vi "configuration UI.vi"() -> ()   [LabVIEW 2013, in "UI Reference editor node.lvclass"]
uses:
  UI Reference editor node.lvclass
  <vilib>/CEF_TreeControl/Node/NodeRef.ctl
  <vilib>/CEF_TreeControl/Node/NISE_CEF_Node.lvclass
  <vilib>/NI/AMC/Message Queue.ctl
  <vilib>/NI/AMC/Message.ctl
  <vilib>/NI/Tools/Keyed Array/KeyedArray.ctl
  <vilib>/CEF_TreeControl/Node/UserEventRef.ctl
  <vilib>/CEF_TreeControl/Controls/EventCluster.ctl
  module/configuration/UI Reference configuration.lvclass
  <vilib>/NI/Module Execution Interface/Engine Configuration/engine configuration.lvclass
  <vilib>/NI/Tag Bus Data Framework/Configuration Editor/Classes/Engine Parent/Engine Parent Editor Node.lvclass
  <vilib>/NI/Tag Bus/tag/tag descriptor.lvclass
  <vilib>/NI/Tag Bus/tag/Data Type.ctl
  <vilib>/NI/Tag Bus/tag/tag descriptor.lvclass/tag descriptor.ctl
  <vilib>/NI/Tag Bus Module Framework/root configuration/TBM configuration.lvclass/TBM configuration.ctl
  module/configuration/UI Reference configuration.lvclass/UI Reference configuration.ctl
  <vilib>/NI/Tag Bus/tag/write tag name.vi
  <vilib>/NI/Tag Bus/tag/write data type.vi
  module/configuration/Read VI Refnum.vi
  module/configuration/Write VI Refnum.vi
  module/configuration/Write VI name.vi
  <vilib>/NI/Tag Bus Module Framework/root configuration/Read instance name.vi
  module/configuration/Read VI name.vi
  <vilib>/NI/Tag Bus Data Framework/Configuration Editor/Classes/Module editor node/Read Module Configuration.vi
  <vilib>/NI/Tag Bus Module Framework/root configuration/create GUID.vi
  <vilib>/NI/Tag Bus Module Framework/root configuration/TBM configuration.lvclass
  <vilib>/NI/Tag Bus Module Framework/module configuration/TBM module configuration.lvclass
  <vilib>/NI/Tag Bus Module Framework/channel/TBM channel.lvclass
  <vilib>/CEF_TreeControl/NISE_CEF_TreeControl.lvlib
  <vilib>/NI/Tag Bus Data Framework/Configuration Editor/Classes/Module editor node/module editor node.lvclass
  <vilib>/NI/Tools/Keyed Array/Tools_KeyedArray.lvlib
  <vilib>/NI/AMC/AMC.lvlib
panel:
  in  "Tab Control":enum32{"Static Configuration"}(tab)
  in  "autogen":bool
  in  "browse":bool
  out "UI to Load":string
  in  "hidden_remove":bool
  in  "hidden_settings":bool
  in  "hidden_Add":bool
  in  "Remove Button":bool
  in  "Add Button":bool
  in  "channel":i32(listbox)
  in  "settings":bool
  in  "user event":T1
  in  "main queue":T2
  in  "node ref":T3
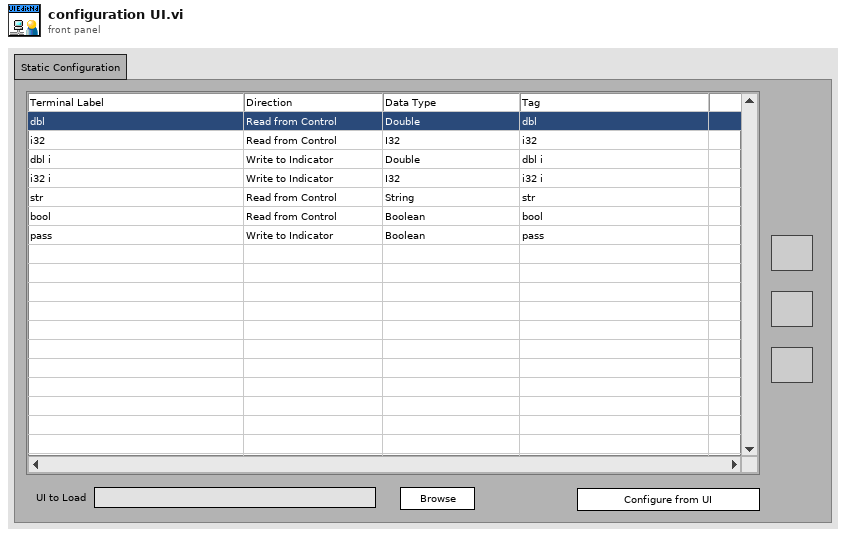
[diagram p1: front panel]
types:
  T1 = typedef "NISE_CEF_Node.lvclass/UserEventRef.ctl" = refnum<user-event>
  T2 = typedef "AMC.lvlib/Message Queue.ctl" = refnum<queue>
  T3 = typedef "NISE_CEF_Node.lvclass/NodeRef.ctl" = refnum<data-value>
  T4 = typedef "tag bus.lvlib/tag descriptor.lvclass/Data Type.ctl" = enum16{"Double", "Single", "I64", "I32", "I16", "I8", "U64", "U32", "U16", "U8", "Boolean", "String", "Array of Double", "Array of Single", "Array of I64", "Array of I32", "Array of I16", "Array of I8", "Array of U64", "Array of U32", "Array of U16", "Array of U8", "Array of Boolean", "Array of String"}
  T5 = typedef "NISE_CEF_TreeControl.lvlib/EventCluster.ctl" = cluster{"command":string, "data":string}
  T6 = typedef "UI Reference editor node.lvclass/table line.ctl" = cluster{"channel":refnum<class "TBM channel.lvclass">, "tag name":string}
  T7 = typedef "LVPoint32TypeDef.ctl" = cluster{"Horizontal":i32, "Vertical":i32}
  T8 = typedef "LVRowAndColumnTypeDef.ctl" = cluster{"Row":i32, "Column":i32}
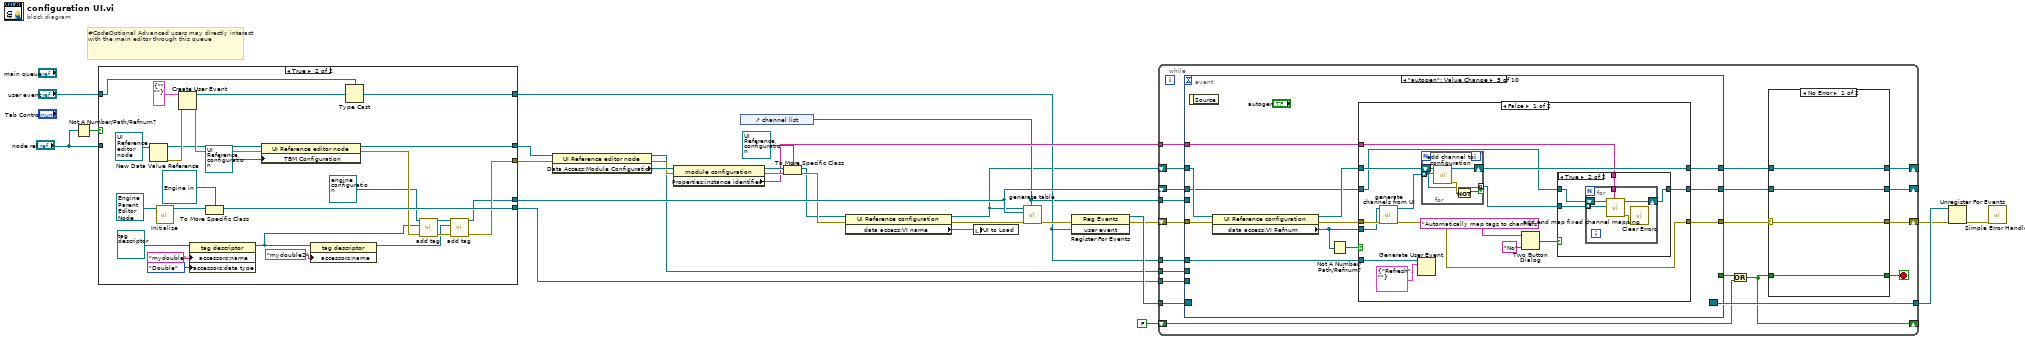
[diagram p0: block diagram]
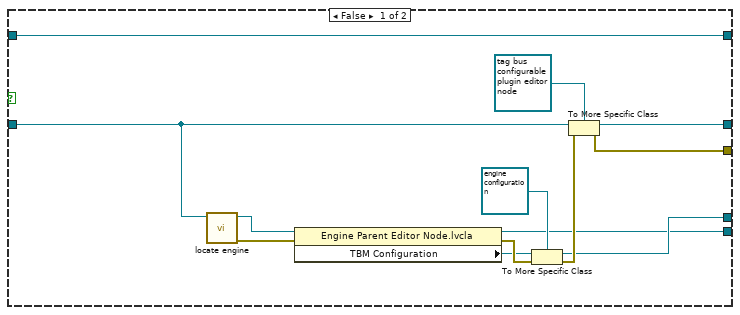
[diagram p2: hidden frame]
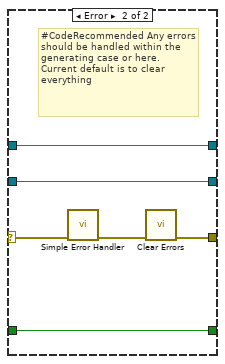
[diagram p3: hidden frame]
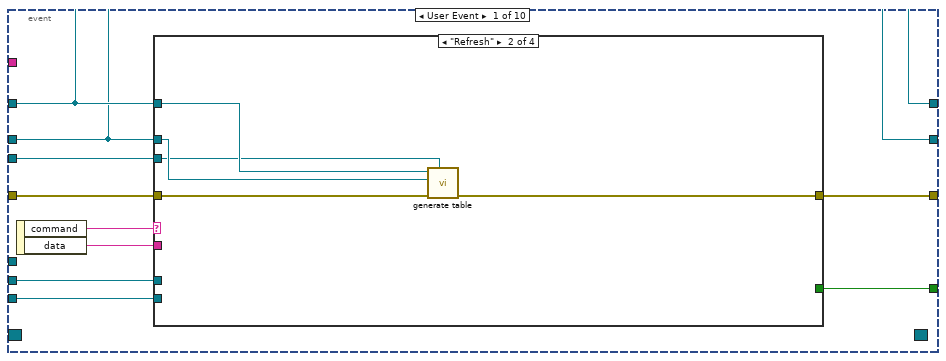
[diagram p4: hidden frame]
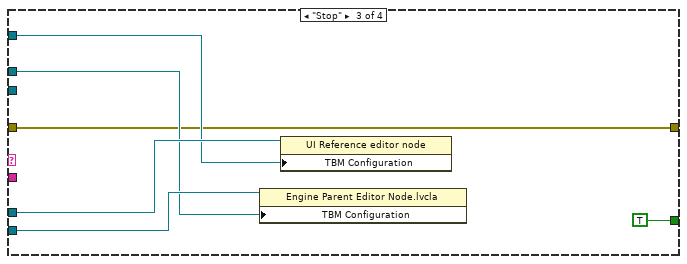
[diagram p6: hidden frame]
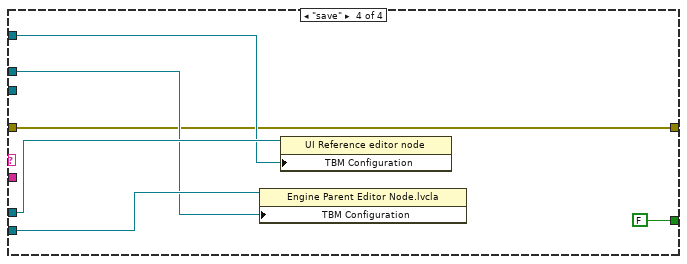
[diagram p7: hidden frame]
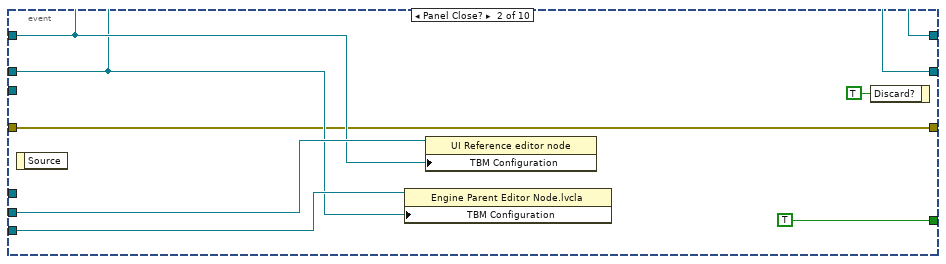
[diagram p8: hidden frame]
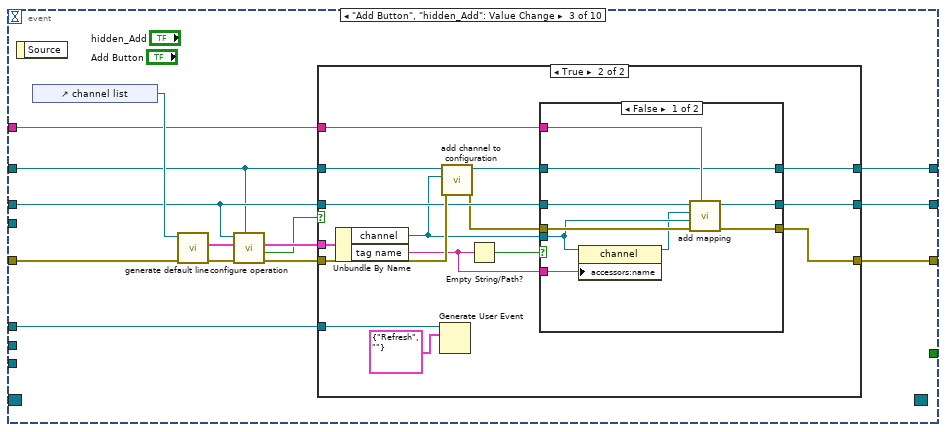
[diagram p9: hidden frame]
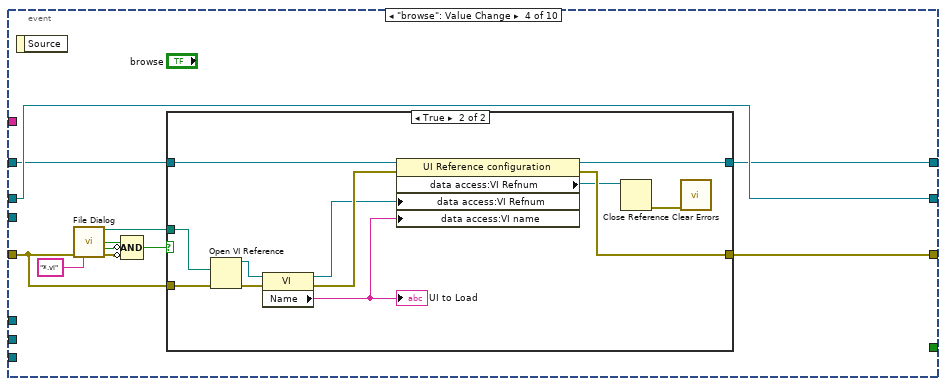
[diagram p12: hidden frame]
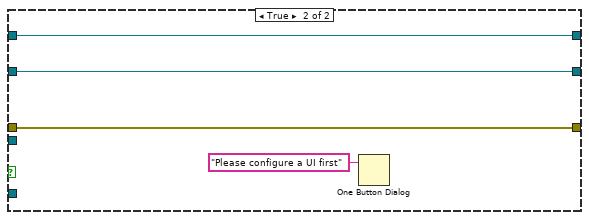
[diagram p15: hidden frame]
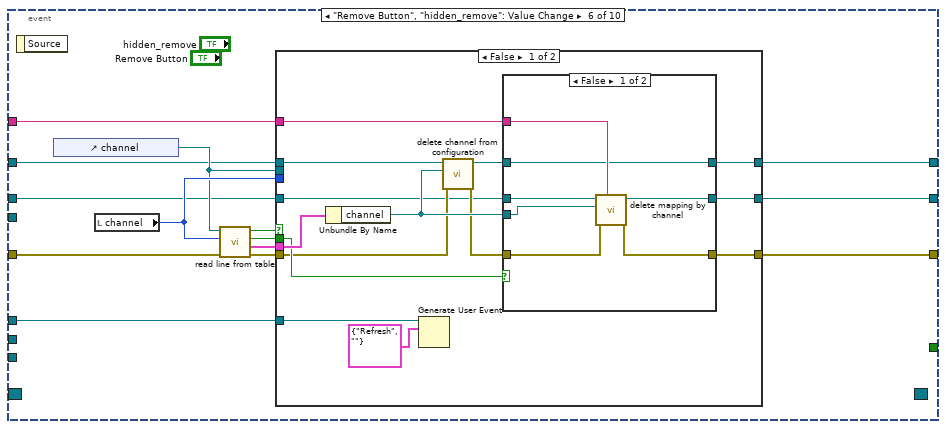
[diagram p16: hidden frame]
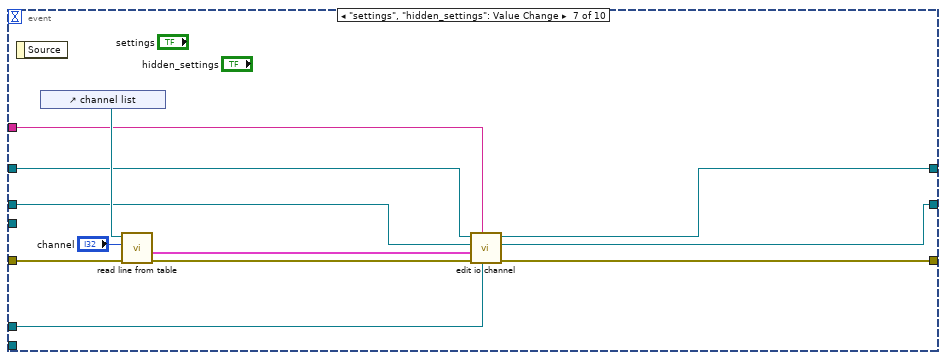
[diagram p19: hidden frame]
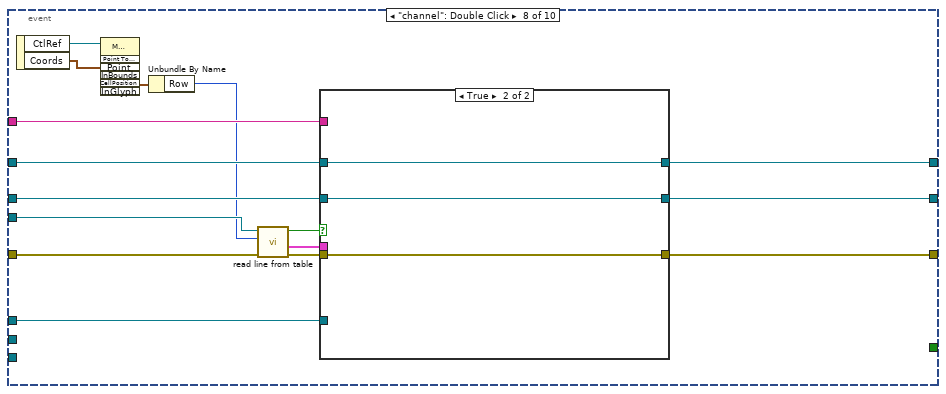
[diagram p20: hidden frame]
diagram:
  # "#CodeOptional Advanced users may directly interact with the main editor through this queue"
  n1 = Not A Number/Path/Refnum?(number/path/refnum="node ref") -> (NaN/Path/Refnum?=w19:bool)
  n2 = case shown="True" w19 {
    tunnel: "user event" -> [w41 w43]
    tunnel: [w41 w44] -> w6
    tunnel: "node ref" -> [w39 _]
    tunnel: [w38 w61] -> w12
    tunnel: [w37 w48] -> w17
    tunnel: [w30 w47] -> w14
    tunnel: [w29 w58] -> w8
    frame False {
      n3 = call <vilib>:"locate engine.vi"("component"=w39) -> ("error out"=w34:errorcluster, "engine"=w36:refnum<data-value>)  [unwired: 9 in]
      n4 = property class="Engine Parent Editor Node.lvcla"(reference=w36, error in=w34) -> (reference out=w29:refnum<data-value>, error out=w33:errorcluster, "TBM Configuration"=w32:refnum<class "TBM configuration.lvclass">)
      n5 = To More Specific Class(target class=refnum<class "engine configuration.lvclass"> refnum ("engine configuration.lvclass"), reference=w32, error in=w33) -> (specific class reference=w30:refnum<class "engine configuration.lvclass">, error out=w31:errorcluster)
      n6 = To More Specific Class(target class=refnum<data-value> refnum ("data value reference"), reference=w39, error in=w31) -> (specific class reference=w38:refnum<data-value>, error out=w37:errorcluster)
    }
    frame True {
      n7 = New Data Value Reference(data value=refnum<class "UI Reference editor node.lvclass"> refnum ("tag bus configurable plugin editor node")) -> (data value reference=w60:refnum<data-value>, error out=w63:errorcluster)  [unwired: 1 in]
      n8 = call-dynamic "Initialize.vi"("Engine in"=refnum<class "Engine Parent Editor Node.lvclass"> refnum) -> ("data value reference"=w59:T3)  [unwired: 8 in, 2 out]
      n9 = Create User Event(user event datatype=T5 {"command"="", "data"=""} ("event data"), error in=w63) -> (user event=w66:refnum<user-event>, error out=w62:errorcluster)
      n10 = property class="tag descriptor"(reference=refnum<class "tag descriptor.lvclass"> refnum ("tag descriptor"), "accessors:name"="mydouble" ("name"), "accessors:data type"=Data_Type."Double" ("data type")) -> (reference out=w45:refnum<class "tag descriptor.lvclass">)  [unwired: 1 in, 1 out]
      n11 = To More Specific Class(target class=refnum<data-value> refnum ("data value reference"), reference=w59) -> (specific class reference=w58:refnum<data-value>)  [unwired: 1 in, 1 out]
      n12 = property class="UI Reference editor node"(reference=w60, error in=w62, "TBM Configuration"=refnum<class "UI Reference configuration.lvclass"> refnum ("tag bus configurable plugin module configuration")) -> (reference out=w61:refnum<data-value>, error out=w52:errorcluster)
      n13 = property class="tag descriptor"(reference=w45, "accessors:name"="mydouble2" ("name")) -> (reference out=w46:refnum<class "tag descriptor.lvclass">)  [unwired: 1 in, 1 out]
      n14 = Type Cast(type=w43, x=w66) -> (*(type *) &x=w44:T1)
      n15 = call <vilib>:"add tag.vi"("error in"=w52, "tag descriptor"=w45, "engine configuration in"=refnum<class "engine configuration.lvclass"> refnum ("Engine Configuration")) -> ("error out"=w50:errorcluster, "engine configuration out"=w49:refnum<class "engine configuration.lvclass">)  [unwired: 7 in]
      n16 = call <vilib>:"add tag.vi"("error in"=w50, "tag descriptor"=w46, "engine configuration in"=w49) -> ("error out"=w48:errorcluster, "engine configuration out"=w47:refnum<class "engine configuration.lvclass">)  [unwired: 7 in]
    }
  }
  n17 = property class="UI Reference editor node"(reference=w12, error in=w17) -> (reference out=w9:refnum<data-value>, error out=w22:errorcluster, "Data Access:Module Configuration"=w23:refnum<class "TBM module configuration.lvclass">)
  n18 = property class="module configuration"(reference=w23, error in=w22) -> (reference out=w20:refnum<class "TBM module configuration.lvclass">, error out=w21:errorcluster, "Properties:instance identifier"=w16:string)
  n19 = control-ref of="channel list"() -> (w5:refnum<vi>)
  n20 = To More Specific Class(target class=refnum<class "UI Reference configuration.lvclass"> refnum ("tag bus configurable plugin module configuration"), reference=w20, error in=w21) -> (specific class reference=w3:refnum<class "UI Reference configuration.lvclass">, error out=w13:errorcluster)
  n21 = property class="UI Reference configuration"(reference=w3, error in=w13) -> (reference out=w2:refnum<class "UI Reference configuration.lvclass">, error out=w4:errorcluster, "data access:VI name"=w1:string)
  n22 = local write "UI to Load"(w1) -> ()
  n23 = call "generate table.vi"("table"=w5, "error in"=w4, "engine configuration"=w14, "tag bus configurable plugin module configuration"=w2) -> ("error out"=w11:errorcluster)  [unwired: 7 in]
  n24 = register-events(error in=w11, w6) -> (reference out=w28:refnum<event-registration>, error out=w10:errorcluster)  [unwired: 1 in]
  n25 = while {
    tunnel: w28 -> [w87]
    tunnel: [w86] -> w27
    shift-right: [w80] -> w26
    shift-left: w10 -> [w85]
    shift-right: [w82] -> _
    shift-left: FALSE -> [w81]
    shift-right: [w76] -> _
    shift-left: w2 -> [w79]
    shift-right: [w77] -> _
    shift-left: w14 -> [w78]
    tunnel: w16 -> [w75]
    tunnel: w9 -> [w72]
    tunnel: w8 -> [w71]
    tunnel: w6 -> [w70]
    tunnel: w5 -> [w68]
    stop <- w84 stop-if-true
    n26 = event shown="[4] \"autogen\": Value Change" {
      selector: w87 -> [_ _ _ _ _ _ _ _ _ _]
      dyn-events: [_ _ _ _ _ _ _ _ _ _] -> w86
      timeout: _ -> [_ _ _ _ _ _ _ _ _ _]
      tunnel: [w107 TRUE _ _ _ _ _ _ _ _] -> w83
      tunnel: [w99 w127 w146 w179 w205 w261 w299 w315 w329 w364] -> w69
      tunnel: w85 -> [w100 w127 w145 w181 w213 w260 w300 w316 w347 w363]
      tunnel: w79 -> [w103 w129 w133 w178 w212 w256 w293 w311 w336 w368]
      tunnel: w78 -> [w102 w128 w134 w187 w207 w255 w294 w312 w332 w367]
      tunnel: [w102 w128 w139 w187 w208 w250 w291 w309 w333 w365] -> w74
      tunnel: [w103 w129 w138 w177 w206 w249 w292 w310 w334 w366] -> w73
      tunnel: w75 -> [_ _ w137 _ w203 w251 w290 w308 _ _]
      tunnel: w72 -> [w105 w131 _ _ _ _ _ _ _ _]
      tunnel: w71 -> [w104 w130 _ _ _ _ _ _ _ _]
      tunnel: w70 -> [_ _ w135 _ w202 w248 w289 w307 _ _]
      tunnel: w68 -> [w98 _ _ _ _ _ _ w306 _ _]
      event User Event {
        n27 = event-data() -> ("command"=w106:string, "data"=w101:string)  [unwired: 1 in]
        n28 = case shown="\"Refresh\"" w106 {
          tunnel: [_ _ TRUE FALSE] -> w107
          tunnel: w105 -> [_ _ w118 w124]
          tunnel: w104 -> [_ _ w117 w123]
          tunnel: w103 -> [_ w113 w116 w122]
          tunnel: w102 -> [_ w112 w115 w121]
          tunnel: w101 -> [_ _ _ _]
          tunnel: w100 -> [w108 w111 w114 w120]
          tunnel: [w108 w110 w114 w120] -> w99
          tunnel: w98 -> [_ w109 _ _]
          frame Default {
          }
          frame "Refresh" {
            n29 = call "generate table.vi"("table"=w109, "error in"=w111, "engine configuration"=w112, "tag bus configurable plugin module configuration"=w113) -> ("error out"=w110:errorcluster)  [unwired: 7 in]
          }
          frame "Stop" {
            n30 = property class="Engine Parent Editor Node.lvcla"(reference=w117, "TBM Configuration"=w115) -> ()  [unwired: 1 in, 2 out]
            n31 = property class="UI Reference editor node"(reference=w118, "TBM Configuration"=w116) -> ()  [unwired: 1 in, 2 out]
          }
          frame "save" {
            n32 = property class="Engine Parent Editor Node.lvcla"(reference=w123, "TBM Configuration"=w121) -> ()  [unwired: 1 in, 2 out]
            n33 = property class="UI Reference editor node"(reference=w124, "TBM Configuration"=w122) -> ()  [unwired: 1 in, 2 out]
          }
        }
      }
      event Panel Close? {
        n34 = event-data() -> ()  [unwired: 1 in, 1 out]
        n35 = property class="Engine Parent Editor Node.lvcla"(reference=w130, "TBM Configuration"=w128) -> ()  [unwired: 1 in, 2 out]
        n36 = property class="UI Reference editor node"(reference=w131, "TBM Configuration"=w129) -> ()  [unwired: 1 in, 2 out]
        n37 = event-data("Discard?"=TRUE) -> ()  [unwired: 1 in, 1 out]
      }
      event "Add Button", "hidden_Add": Value Change {
        n38 = event-data() -> ()  [unwired: 1 in, 1 out]
        n39 = control-ref of="channel list"() -> (w144:refnum<vi>)
        n40 = call "generate default line.vi"("error in"=w145, "operations table"=w144) -> ("error out"=w142:errorcluster, "line"=w143:T6)  [unwired: 8 in]
        n41 = call "configure operation.vi"("tag bus configurable plugin module configuration"=w133, "error in"=w142, "line item in"=w143, "engine configuration"=w134) -> ("error out"=w140:errorcluster, "success"=w136:bool, "line item out"=w141:T6)  [unwired: 4 in, 1 out]
        n42 = case shown="True" w136 {
          tunnel: [w149 w152] -> w146
          tunnel: w140 -> [w149 w162]
          tunnel: w134 -> [w148 w160]
          tunnel: w141 -> [_ w163]
          tunnel: w133 -> [w147 w164]
          tunnel: [w148 w159] -> w139
          tunnel: [w147 w153] -> w138
          tunnel: w137 -> [_ w156]
          tunnel: w135 -> [_ w151]
          frame False {
          }
          frame True {
            n43 = Unbundle By Name(w163) -> ("channel"=w157:refnum<class "TBM channel.lvclass">, "tag name"=w155:string)
            n44 = Generate User Event(user event=w151, event data cluster=T5 {"command"="Refresh", "data"=""} ("event data")) -> ()  [unwired: 2 in, 2 out]
            n45 = call "add channel to configuration.vi"("error in"=w162, "channel"=w157, "UI Reference configuration in"=w164) -> ("error out"=w158:errorcluster, "UI Reference configuration out"=w154:refnum<class "UI Reference configuration.lvclass">)  [unwired: 7 in]
            n46 = Empty String/Path?(string/path=w155) -> (empty?=w161:bool)
            n47 = case shown="False" w161 {
              tunnel: w160 -> [w173 w176]
              tunnel: [w172 w176] -> w159
              tunnel: w158 -> [w171 w175]
              tunnel: w157 -> [w169 _]
              tunnel: w156 -> [w170 _]
              tunnel: w155 -> [w168 _]
              tunnel: [w166 w175] -> w152
              tunnel: w154 -> [w165 w174]
              tunnel: [w165 w174] -> w153
              frame False {
                n48 = property class="channel"(reference=w169, "accessors:name"=w168) -> (reference out=w167:refnum<class "TBM channel.lvclass">)  [unwired: 1 in, 1 out]
                n49 = call <vilib>:"add mapping.vi"("owner ID"=w170, "error in"=w171, "channel"=w169, "tag descriptor"=w167, "engine configuration"=w173) -> ("error out"=w166:errorcluster, "engine configuration out"=w172:refnum<class "engine configuration.lvclass">)  [unwired: 5 in]
              }
              frame True {
              }
            }
          }
        }
      }
      event "browse": Value Change {
        n50 = event-data() -> ()  [unwired: 1 in, 1 out]
        n51 = call "File Dialog"("error in"=w181, "pattern (all files)"="*.vi") -> ("selected path"=w180:path, "exists"=w185:bool, "cancelled"=w184:bool, "error out"=w183:errorcluster)  [unwired: 10 in]
        n52 = Compound Arithmetic op=AND(w185, invert w184, invert w183) -> (w182:bool)
        n53 = case shown="True" w182 {
          tunnel: w181 -> [w189 w201]
          tunnel: w180 -> [_ w200]
          tunnel: [w189 w192] -> w179
          tunnel: w178 -> [w188 w197]
          tunnel: [w188 w196] -> w177
          frame False {
          }
          frame True {
            n54 = Open VI Reference(vi path=w200, error in (no error)=w201) -> (vi reference=w198:refnum<vi>, error out=w199:errorcluster)  [unwired: 4 in]
            n55 = property class="VI"(reference=w198, error in=w199) -> (reference out=w193:refnum<vi>, error out=w195:errorcluster, "Name"=w194:string)
            "UI to Load" <- w194
            n56 = property class="UI Reference configuration"(reference=w197, error in=w195, "data access:VI Refnum"=w193, "data access:VI name"=w194) -> (reference out=w196:refnum<class "UI Reference configuration.lvclass">, error out=w192:errorcluster, "data access:VI Refnum"=w191:refnum<vi>)
            n57 = Close Reference(reference=w191) -> (error out=w190:errorcluster)  [unwired: 1 in]
            n58 = call <vilib>:"Clear Errors.vi"("error in (no error)"=w190) -> ()  [unwired: 6 in, 1 out]
          }
        }
      }
      event "autogen": Value Change {
        n59 = event-data() -> ()  [unwired: 1 in, 1 out]
        n60 = property class="UI Reference configuration"(reference=w212, error in=w213) -> (reference out=w209:refnum<class "UI Reference configuration.lvclass">, error out=w210:errorcluster, "data access:VI Refnum"=w204:refnum<vi>)
        n61 = Not A Number/Path/Refnum?(number/path/refnum=w204) -> (NaN/Path/Refnum?=w211:bool)
        n62 = case shown="False" w211 {
          tunnel: w210 -> [w228 w245]
          tunnel: w209 -> [w226 w246]
          tunnel: [w219 w247] -> w208
          tunnel: w207 -> [w220 w247]
          tunnel: [w221 w246] -> w206
          tunnel: [w217 w245] -> w205
          tunnel: w204 -> [w227 _]
          tunnel: w203 -> [w216 _]
          tunnel: w202 -> [w214 _]
          frame False {
            n63 = call "generate channels from UI.vi"("error in"=w228, "VI Refnum"=w227) -> ("error out"=w217:errorcluster, "channels"=w225:refnum<class "TBM channel.lvclass">[])  [unwired: 8 in]
            n64 = Generate User Event(user event=w214, event data cluster=T5 {"command"="Refresh", "data"=""} ("event data")) -> ()  [unwired: 2 in, 2 out]
            n65 = for {
              tunnel: w225 -> [w240] mode=indexing
              shift-right: [w242] -> w221
              shift-left: w226 -> [w243]
              tunnel: [w240] -> w218 mode=indexing if=w239
              n66 = call "add channel to configuration.vi"("channel"=w240, "UI Reference configuration in"=w243) -> ("error out"=w241:errorcluster, "UI Reference configuration out"=w242:refnum<class "UI Reference configuration.lvclass">)  [unwired: 8 in]
              n67 = Not(x=w241) -> (.not. x?=w239:bool)
            }
            n68 = Two Button Dialog(message="Automatically map tags to channels?", 1:"No" ("F button name (\"Cancel\")")) -> (T button?=w222:bool)  [unwired: 1 in]
            n69 = case shown="True" w222 {
              tunnel: w220 -> [w229 w233]
              tunnel: [w229 w232] -> w219
              tunnel: w218 -> [_ w231]
              tunnel: w216 -> [_ w230]
              frame False {
              }
              frame True {
                n70 = for {
                  shift-right: [w237] -> w232
                  shift-left: w233 -> [w238]
                  tunnel: w231 -> [w236] mode=indexing
                  tunnel: w230 -> [w234]
                  n71 = call <vilib>:"add and map fixed channel mapping.vi"("module instance"=w234, "fixed channel"=w236, "engine configuration in"=w238) -> ("error out"=w235:errorcluster, "engine configuration out"=w237:refnum<class "engine configuration.lvclass">)  [unwired: 7 in]
                  n72 = call <vilib>:"Clear Errors.vi"("error in (no error)"=w235) -> ()  [unwired: 6 in, 1 out]
                }
              }
            }
          }
          frame True {
            n73 = One Button Dialog(message="Please configure a UI first") -> ()  [unwired: 1 in, 1 out]
          }
        }
      }
      event "Remove Button", "hidden_remove": Value Change {
        n74 = event-data() -> ()  [unwired: 1 in, 1 out]
        n75 = control-ref of="channel"() -> (w258:refnum<vi>)
        n76 = local read "channel"() -> (w259:i32)
        n77 = call "read line from table.vi"("error in"=w260, "line number"=w259, "channels table"=w258) -> ("error out"=w252:errorcluster, "line"=w257:T6, "empty tag?"=w253:bool, "empty channel?"=w254:bool)  [unwired: 5 in]
        n78 = case shown="False" w254 {
          tunnel: [w264 w287] -> w261
          tunnel: w259 -> [_ _]
          tunnel: w258 -> [_ _]
          tunnel: w257 -> [w275 _]
          tunnel: w256 -> [w273 w286]
          tunnel: w255 -> [w268 w288]
          tunnel: w253 -> [w274 _]
          tunnel: w252 -> [w271 w287]
          tunnel: w251 -> [w267 _]
          tunnel: [w266 w288] -> w250
          tunnel: [w265 w286] -> w249
          tunnel: w248 -> [w262 _]
          frame False {
            n79 = Unbundle By Name(w275) -> ("channel"=w272:refnum<class "TBM channel.lvclass">)
            n80 = Generate User Event(user event=w262, event data cluster=T5 {"command"="Refresh", "data"=""} ("event data")) -> ()  [unwired: 2 in, 2 out]
            n81 = call "delete channel from configuration.vi"("error in"=w271, "channel"=w272, "UI Reference configuration in"=w273) -> ("error out"=w269:errorcluster, "UI Reference configuration out"=w270:refnum<class "UI Reference configuration.lvclass">)  [unwired: 7 in]
            n82 = case shown="False" w274 {
              tunnel: w272 -> [w281 _]
              tunnel: w270 -> [w276 w283]
              tunnel: w269 -> [w279 w284]
              tunnel: w268 -> [w282 w285]
              tunnel: w267 -> [w280 _]
              tunnel: [w278 w285] -> w266
              tunnel: [w277 w284] -> w264
              tunnel: [w276 w283] -> w265
              frame False {
                n83 = call <vilib>:"delete mapping by channel.vi"("owner ID"=w280, "error in"=w279, "channel"=w281, "engine configuration in"=w282) -> ("error out"=w277:errorcluster, "engine configuration out"=w278:refnum<class "engine configuration.lvclass">)  [unwired: 6 in]
              }
              frame True {
              }
            }
          }
          frame True {
          }
        }
      }
      event "settings", "hidden_settings": Value Change {
        n84 = event-data() -> ()  [unwired: 1 in, 1 out]
        n85 = control-ref of="channel list"() -> (w298:refnum<vi>)
        n86 = call "read line from table.vi"("error in"=w300, "line number"="channel", "channels table"=w298) -> ("error out"=w297:errorcluster, "line"=w296:T6)  [unwired: 5 in, 2 out]
        n87 = call "edit io channel.vi"("user event"=w289, "Properties:instance identifier"=w290, "error in"=w297, "line"=w296, "engine configuration in"=w294, "tag bus configurable plugin module configuration in"=w293) -> ("error out"=w299:errorcluster, "engine configuration"=w291:refnum<class "engine configuration.lvclass">, "tag bus configurable plugin module configuration out"=w292:refnum<class "UI Reference configuration.lvclass">)  [unwired: 3 in]
      }
      event "channel": Double Click {
        n88 = event-data() -> ("CtlRef"=w305:refnum<vi>, "Coords"=w304:T7)  [unwired: 1 in]
        n89 = invoke class="MCListbox (strict)" method="Point To Row Column"(reference=w305, "Point"=w304) -> ("CellPosition"=w303:T8)  [unwired: 5 in, 6 out]
        n90 = Unbundle By Name(w303) -> ("Row"=w302:i32)
        n91 = call "read line from table.vi"("error in"=w316, "line number"=w302, "channels table"=w306) -> ("error out"=w314:errorcluster, "line"=w313:T6, "empty channel?"=w301:bool)  [unwired: 5 in, 1 out]
        n92 = case shown="True" w301 {
          tunnel: [w325 w326] -> w315
          tunnel: w314 -> [w324 w326]
          tunnel: w313 -> [w323 _]
          tunnel: w312 -> [w322 w327]
          tunnel: w311 -> [w321 w328]
          tunnel: [w320 w328] -> w310
          tunnel: [w319 w327] -> w309
          tunnel: w308 -> [w318 _]
          tunnel: w307 -> [w317 _]
          frame False {
            n93 = call "edit io channel.vi"("user event"=w317, "Properties:instance identifier"=w318, "error in"=w324, "line"=w323, "engine configuration in"=w322, "tag bus configurable plugin module configuration in"=w321) -> ("error out"=w325:errorcluster, "engine configuration"=w319:refnum<class "engine configuration.lvclass">, "tag bus configurable plugin module configuration out"=w320:refnum<class "UI Reference configuration.lvclass">)  [unwired: 3 in]
          }
          frame True {
          }
        }
      }
      event "channel": Shortcut Menu Activation? {
        n94 = event-data() -> ("MenuRef"=w343:refnum<k9>, "CtlRef"=w345:refnum<vi>, "Coords"=w344:T7)  [unwired: 1 in]
        n95 = invoke class="MCListbox (strict)" method="Point To Row Column"(reference=w345, "Point"=w344) -> (reference out=w342:refnum<vi>, error out=w341:errorcluster, "CellPosition"=w340:T8)  [unwired: 5 in, 4 out]
        n96 = Delete Menu Items(6:w347, 9:w343) -> (0:w330:errorcluster, 3:w331:refnum<k9>)  [unwired: 2 in]
        n97 = Unbundle(w340) -> ("Row"=w338:i32)  [unwired: 1 out]
        n98 = property class="MCListbox (strict)"(reference=w342, error in=w341) -> ("ItemNames"=w339:string[][])  [unwired: 2 out]
        n99 = Index Array(array=w339, index (row)=w338, index (col)=0 ("disabled index (col)")) -> (element=w335:string)
        n100 = case shown="\"\"" w335 {
          tunnel: w336 -> [w353 w359]
          tunnel: [w353 w359] -> w334
          tunnel: [w352 w358] -> w333
          tunnel: w332 -> [w352 w358]
          tunnel: w331 -> [w351 w357]
          tunnel: w330 -> [w350 w356]
          tunnel: [w349 w355] -> w329
          frame Default {
            w348 = string[] ["Add", "Edit", "Delete"] ("item names")
            n101 = Insert Menu Items(6:w350, 7:w348, 8:w348, 9:w351) -> (0:w349:errorcluster)  [unwired: 2 in, 2 out]
          }
          frame "" {
            w354 = string[] ["Add"] ("item names")
            n102 = Insert Menu Items(6:w356, 7:w354, 8:w354, 9:w357) -> (0:w355:errorcluster)  [unwired: 2 in, 2 out]
          }
        }
        n103 = event-data("Discard?"=FALSE) -> ()  [unwired: 1 in, 1 out]
      }
      event "channel": Shortcut Menu Selection (User) {
        n104 = event-data() -> ("ItemTag"=w369:string, "CtlRef"=w370:refnum<vi>, "Coords"=w371:T7)  [unwired: 1 in]
        n105 = invoke class="MCListbox (strict)" method="Point To Row Column"(reference=w370, "Point"=w371) -> ("CellPosition"=w361:T8)  [unwired: 5 in, 6 out]
        n106 = Unbundle By Name(w361) -> ("Row"=w360:i32)
        n107 = property on="channel" class="MCListbox (strict)"(error in=w363, "Value"=w360) -> (error out=w362:errorcluster)  [unwired: 1 in, 1 out]
        n108 = case shown="\"Delete\"" w369 {
          tunnel: w362 -> [w372 w376 w382 w387]
          tunnel: w368 -> [w374 w379 w384 w389]
          tunnel: w367 -> [w373 w378 w383 w388]
          tunnel: [w374 w379 w384 w389] -> w366
          tunnel: [w373 w378 w383 w388] -> w365
          tunnel: [w372 w375 w381 w386] -> w364
          frame Default {
          }
          frame "Add" {
            n109 = property on="hidden_Add" class="Bool (strict)"(error in=w376, "Val(Sgnl)"=TRUE ("Value (Signaling)")) -> (error out=w375:errorcluster)  [unwired: 1 in, 1 out]
          }
          frame "Edit" {
            n110 = property on="hidden_settings" class="Bool (strict)"(error in=w382, "Val(Sgnl)"=TRUE ("Value (Signaling)")) -> (error out=w381:errorcluster)  [unwired: 1 in, 1 out]
          }
          frame "Delete" {
            n111 = property on="hidden_remove" class="Bool (strict)"(error in=w387, "Val(Sgnl)"=FALSE ("Value (Signaling)")) -> (error out=w386:errorcluster)  [unwired: 1 in, 1 out]
          }
        }
      }
    }
    n112 = Or(x=w83, y=w81) -> (x .or. y?=w82:bool)
    n113 = case shown="No Error" w69 {
      selector: w69 -> [w88 w96]
      tunnel: [w91 w97] -> w84
      tunnel: w82 -> [w91 w97]
      tunnel: [w88 w94] -> w80
      tunnel: w74 -> [w89 w93]
      tunnel: [w89 w93] -> w77
      tunnel: w73 -> [w90 w92]
      tunnel: [w90 w92] -> w76
      frame No Error {
      }
      frame Error {
        # "#CodeRecommended Any errors should be handled within the generating case or here. Current default is to clear everything"
        n114 = call <vilib>:"Simple Error Handler.vi"("error in (no error)"=w96) -> ("error out"=w95:errorcluster)  [unwired: 4 in, 4 out]
        n115 = call <vilib>:"Clear Errors.vi"("error in (no error)"=w95) -> ("error out"=w94:errorcluster)  [unwired: 6 in]
      }
    }
  }
  n116 = Unregister For Events(event registration refnum=w27, error in=w26) -> (error out=w7:errorcluster)
  n117 = call <vilib>:"Simple Error Handler.vi"("error in (no error)"=w7) -> ()  [unwired: 4 in, 5 out]
